vi "Solenoid Globals.vi"() -> ()   [LabVIEW 2019]
panel:
  in  "Control_Panel_Pneumatic":string="Control_Panel_Pneumatic"
  in  "Climb_Lock":string="Climb_Lock"
  in  "Intake_Extend_And_Retract":string="Intake_Extend_And_Retract"
  in  "Compressor":string="Compressor"
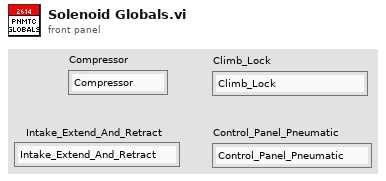
[diagram p1: front panel]
diagram:
